vi "23_1b.vi"() -> ()   [LabVIEW 2020]
uses:
  <vilib>/Analysis/1siggen.llb/Ramp Pattern by Delta.vi
  <vilib>/Analysis/NI_AALBase.lvlib
panel:
  out "concatenated string":string="69852437"
  out "Previous":i32[](array[numeric])=[3, 9, 8, 5, 7, 1, 6, 2, 4]
  out "Current Cup":i32=6
  out "Pickup":i32[](array[numeric])=[2, 4, 3]
  out "Destination Cup":i32=5
  out "Next Cup":i32=9
  out "Array":i32[](array[numeric])=[5, 2, 4, 3, 7, 1, 6, 9, 8]
  in  "Moves":i32=100
  in  "Switch":bool
  in  "Input":string="925176834"
  in  "Input Test":string="389125467"
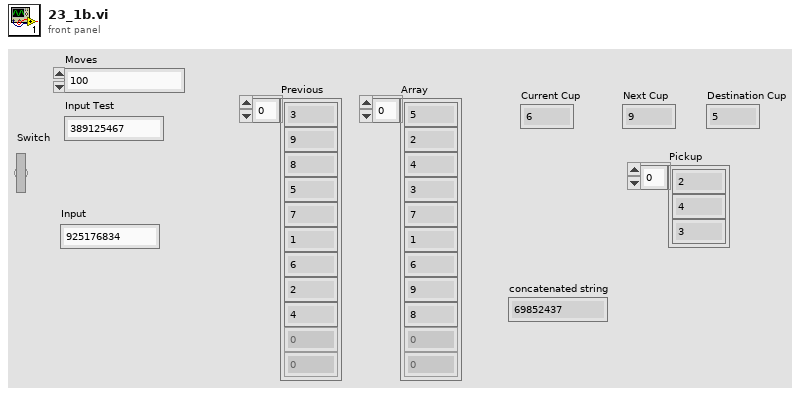
[diagram p1: front panel]
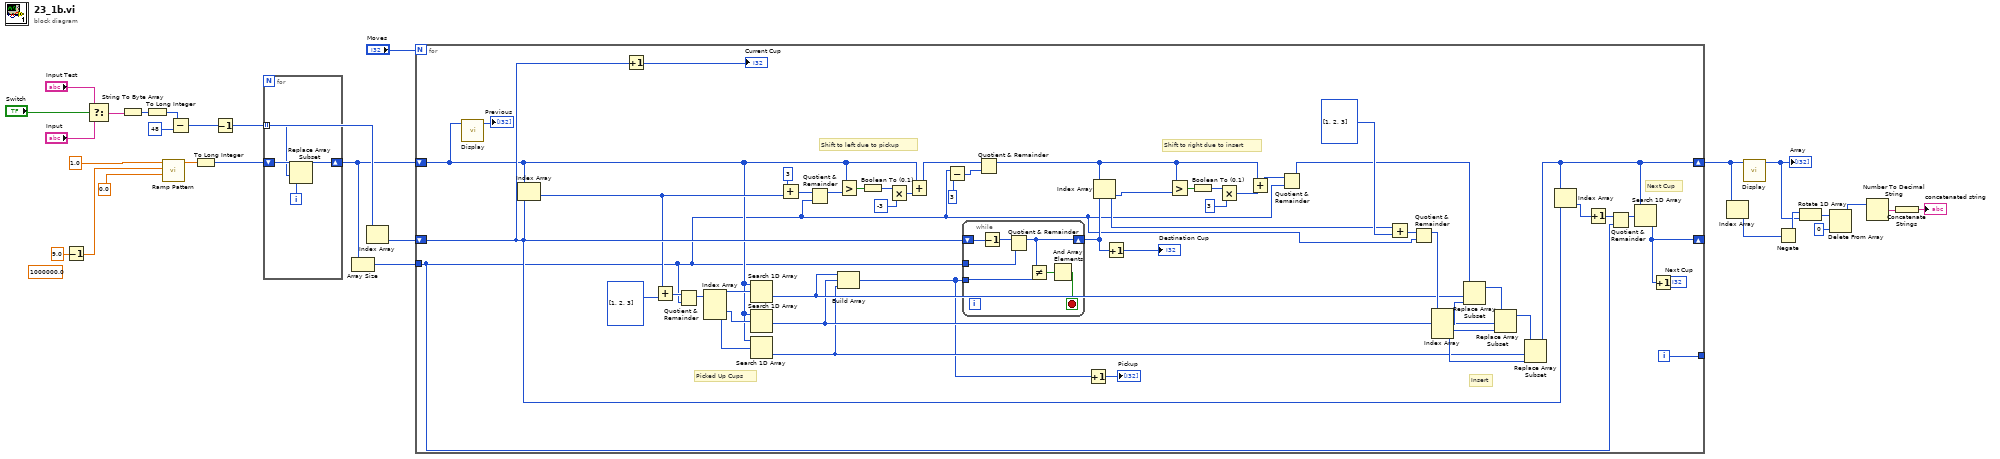
[diagram p0: block diagram]
diagram:
  (unwired) 1000000.0 ("end")
  n1 = Decrement(x=9.0 ("end")) -> (x-1=w16:dbl)
  n2 = Select(t="Input Test", s="Switch", f="Input") -> (s? t:f=w25:string)
  n3 = String To Byte Array(string=w25) -> (unsigned byte array=w24:u8[])
  n4 = To Long Integer(number=w24) -> (32bit integer=w21:i32[])
  n5 = call-poly <vilib>:"Ramp Pattern.vi"("start"=0.0, "end"=w16, "delta"=1.0) -> ("Ramp Pattern"=w18:dbl[])  [unwired: 6 in, 2 out]
  n6 = Subtract(x=w21, y=48) -> (x-y=w15:i32[])
  n7 = To Long Integer(number=w18) -> (32bit integer=w11:i32[])
  n8 = Decrement(x=w15) -> (x-1=w13:i32[])
  n9 = for {
    tunnel: w13 -> [w30] mode=indexing
    shift-right: [w29] -> w10
    shift-left: w11 -> [w32]
    i -> [w31]
    n10 = Replace Array Subset(array=w32, new element=w31, index=w30) -> (w29:i32[])
  }
  n11 = Array Size(array=w10) -> (size(s)=w14:i32)
  n12 = Index Array(array=w13) -> (element=w12:i32)  [unwired: 1 in]
  n13 = for {
    N: "Moves" -> [_]
    shift-right: [w42] -> w9
    shift-left: w10 -> [w38]
    tunnel: [w84] -> _
    shift-right: [w49] -> _
    shift-left: w12 -> [w41]
    tunnel: w14 -> [w35]
    i -> [w84]
    # "Picked Up Cups"
    # "Next Cup"
    # "Insert"
    # "Shift to right due to insert"
    # "Shift to left due to pickup"
    n14 = call "Display.vi"("Array in"=w38) -> ("Array out"=→"Previous":i32[])  [unwired: 10 in]
    n15 = Index Array(array=w38, index=w41) -> (element=w40:i32)
    n16 = Increment(x=w41) -> (x+1=→"Current Cup":i32)
    n17 = Add(x=w40, y=i32[] [1, 2, 3]) -> (x+y=w71:i32[])
    n18 = Quotient & Remainder(x=w71, y=w35) -> (x-y*floor(x/y)=w70:i32[])  [unwired: 1 out]
    n19 = Index Array(array=w70) -> (element #1=w69:i32, element #2=w68:i32, element #3=w67:i32)  [unwired: 3 in]
    n20 = Search 1D Array(1D array=w38, element=w69) -> (index of element=w52:i32)  [unwired: 1 in]
    n21 = Search 1D Array(1D array=w38, element=w68) -> (index of element=w51:i32)  [unwired: 1 in]
    n22 = Search 1D Array(1D array=w38, element=w67) -> (index of element=w50:i32)  [unwired: 1 in]
    n23 = Add(x=3, y=w40) -> (x+y=w73:i32)
    n24 = Quotient & Remainder(x=w73, y=w35) -> (x-y*floor(x/y)=w58:i32)  [unwired: 1 out]
    n25 = Greater?(x=w38, y=w58) -> (0:w83:bool[])
    n26 = Build Array(w52, w51, w50) -> (w45:i32[])
    n27 = Boolean To (0,1)(Boolean=w83) -> (0, 1=w82:i16[])
    n28 = Multiply(x=w82, y=-3) -> (x*y=w80:i32[])
    n29 = Add(x=w38, y=w80) -> (x+y=w57:i32[])
    n30 = Subtract(x=w35, y=3) -> (x-y=w34:i32)
    n31 = while {
      tunnel: w35 -> [w89]
      shift-right: [w88] -> w47
      shift-left: w41 -> [w91]
      tunnel: w45 -> [w87]
      stop <- w85 stop-if-true
      n32 = Decrement(x=w91) -> (x-1=w90:i32)
      n33 = Quotient & Remainder(x=w90, y=w89) -> (x-y*floor(x/y)=w88:i32)  [unwired: 1 out]
      n34 = Not Equal?(x=w88, y=w87) -> (x != y?=w86:bool[])
      n35 = And Array Elements(Boolean array=w86) -> (logical AND=w85:bool)
    }
    n36 = Quotient & Remainder(x=w57, y=w34) -> (x-y*floor(x/y)=w54:i32[])  [unwired: 1 out]
    n37 = Increment(x=w45) -> (x+1=→"Pickup":i32[])
    n38 = Index Array(array=w54, index=w47) -> (element=w36:i32)
    n39 = Increment(x=w47) -> (x+1=→"Destination Cup":i32)
    n40 = Greater?(x=w54, y=w36) -> (0:w76:bool[])
    n41 = Boolean To (0,1)(Boolean=w76) -> (0, 1=w77:i16[])
    n42 = Multiply(x=w77, y=3) -> (x*y=w79:i32[])
    n43 = Add(x=w54, y=w79) -> (x+y=w56:i32[])
    n44 = Quotient & Remainder(x=w56, y=w35) -> (x-y*floor(x/y)=w53:i32[])  [unwired: 1 out]
    n45 = Add(x=w36, y=i32[] [1, 2, 3]) -> (x+y=w64:i32[])
    n46 = Quotient & Remainder(x=w64, y=w35) -> (x-y*floor(x/y)=w62:i32[])  [unwired: 1 out]
    n47 = Index Array(array=w62) -> (element #1=w61:i32, element #2=w60:i32, element #3=w59:i32)  [unwired: 3 in]
    n48 = Replace Array Subset(array=w53, new element=w61, index=w52) -> (w66:i32[])
    n49 = Replace Array Subset(array=w66, new element=w60, index=w51) -> (w65:i32[])
    n50 = Replace Array Subset(array=w65, new element=w59, index=w50) -> (w42:i32[])
    n51 = Index Array(array=w42, index=w41) -> (element=w39:i32)
    n52 = Increment(x=w39) -> (x+1=w75:i32)
    n53 = Quotient & Remainder(x=w75, y=w35) -> (x-y*floor(x/y)=w74:i32)  [unwired: 1 out]
    n54 = Search 1D Array(1D array=w42, element=w74) -> (index of element=w49:i32)  [unwired: 1 in]
    n55 = Increment(x=w49) -> (x+1=→"Next Cup":i32)
  }
  n56 = Index Array(array=w9) -> (element=w2:i32)  [unwired: 1 in]
  n57 = call "Display.vi"("Array in"=w9) -> ("Array out"=w3:i32[])  [unwired: 10 in]
  "Array" <- w3
  n58 = Negate(x=w2) -> (-x=w6:i32)
  n59 = Rotate 1D Array(1:w3, 2:w6) -> (0:w5:i32[])
  n60 = Delete From Array(array=w5, index=0) -> (array with subset deleted=w1:i32[])  [unwired: 1 in, 1 out]
  n61 = Number To Decimal String(number=w1) -> (decimal integer string=w8:string[])  [unwired: 1 in]
  n62 = Concatenate Strings(w8) -> (→"concatenated string":string)
